vi "Topic Actor.vi"(9 "Inbox":refnum<class "Message Transport Queue.lvclass">, 10 "Topic Name":string, 11 "Topic Actor in":refnum<class "Topic Actor.lvclass">) -> ()   [LabVIEW 2016, in "Stream Mediator.lvlib" / "Topic Actor.lvclass"]
doc: "--\nCopyright © 2017 Composed SystemsI All rights reserved.\n\nAuthor: Jon McBee <jon.mcbee@composed.io>\n\nThis library is provided \"AS IS\" ,WITHOUT WARRANTIES OR\nCONDITIONS OF ANY KIND, either express or implied.\n\nComposed Systems -- composed.io\n\nStream 0.0.1.1\nJon McBee - Composed Systems\nCopyright (c) 2017, Composed Systems"
uses:
  <userlib>/Composed Systems/Stream/Mediator/Classes/Topic Actor/Topic Actor.lvclass
  <userlib>/Composed Systems/Stream/Mediator/Classes/Message Transport Queue/Message Transport Queue.lvclass
  <userlib>/Composed Systems/Stream/Mediator/Classes/Subscriber Look Up Table/Subscriber Look Up Table.lvclass
  <userlib>/Composed Systems/Stream/Mediator/Classes/Topic Actor/Topic Actor.lvclass/Topic Actor.ctl
panel:
  out "Topic Actor out":refnum<class "Topic Actor.lvclass">
  out "error out":errorcluster
  in  "error in (no error)":errorcluster
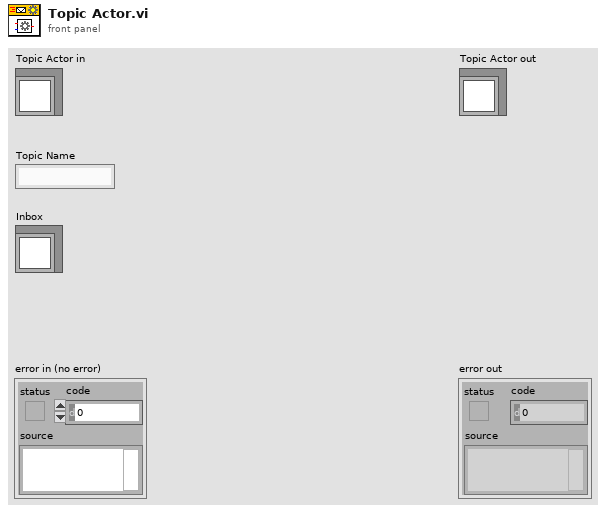
[diagram p1: front panel]
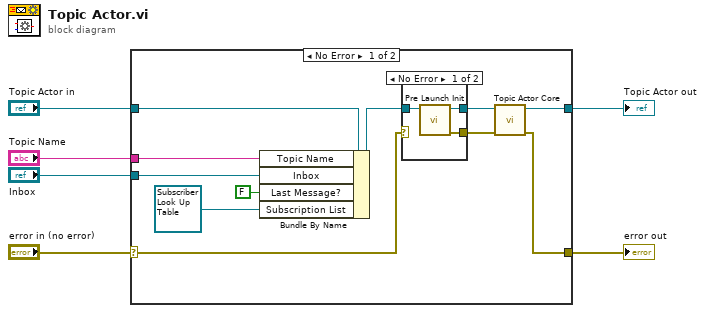
[diagram p0: block diagram]
diagram:
  n1 = case shown="No Error" "error in (no error)" {
    selector: "error in (no error)" -> [w8 w24]
    tunnel: [w12 w24] -> w5
    tunnel: [w13 w23] -> w3
    tunnel: "Topic Actor in" -> [w17 w23]
    tunnel: "Topic Name" -> [w16 _]
    tunnel: "Inbox" -> [w15 _]
    frame No Error {
      n2 = Bundle By Name(cluster=w17, "Topic Name"=w16, "Inbox"=w15, "Last Message?"=FALSE, "Subscription List"=refnum<class "Subscriber Look Up Table.lvclass"> refnum) -> (w10:refnum<class "Topic Actor.lvclass">)
      n3 = case shown="No Error" w8 {
        selector: w8 -> [_ w22]
        tunnel: w10 -> [w20 w21]
        tunnel: [w19 w21] -> w9
        tunnel: [w18 w22] -> w7
        frame No Error {
          n4 = call-dynamic "Pre Launch Init.vi"("Topic Actor in"=w20) -> ("error out"=w18:errorcluster, "Topic Actor out"=w19:refnum<class "Topic Actor.lvclass">)  [unwired: 9 in]
        }
        frame Error {
        }
      }
      n5 = call-dynamic "Topic Actor Core.vi"("error in (no error)"=w7, "Topic Actor in"=w9) -> ("error out"=w12:errorcluster, "Topic Actor out"=w13:refnum<class "Topic Actor.lvclass">)  [unwired: 8 in]
    }
    frame Error {
    }
  }
  "error out" <- w5
  "Topic Actor out" <- w3
